vi "Write Ack.vi"(10 "id":u32) -> (2 "channel":T1)   [LabVIEW 2019, in "MessengerM.lvlib"]
doc: "Writes an acknowledgement to a Messenger channel that the message with the given id has been read."
uses:
  <resource>/Channels/MessengerM/MessengerM.lvlib
  <resource>/Channels/MessengerM/EndpointOp.ctl
  <resource>/Channels/MessengerM/ParmsIn.ctl
  <resource>/Channels/MessengerM/))Channel.ctl
  <resource>/Channels/MessengerM/Element.ctl
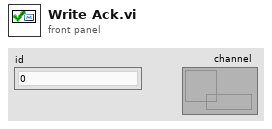
[diagram p1: front panel]
types:
  T1 = typedef "MessengerM.lvlib/))Channel.ctl" = refnum<queue>
  T2 = typedef "MessengerM.lvlib/ParmsIn.ctl" = cluster{"subchannel":i32, "size (0)":i32, "abort (F)":bool, "timeout":i32, "ack id (0)":u32, "last elt? (F)":bool, "valid? (T)":bool, "GUID":string}
  T3 = typedef "MessengerM.lvlib/EndpointOp.ctl" = enum16{"Write", "WriteAck", "WriteSync", "Read", "ReadAck"}
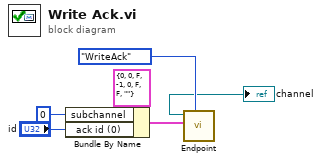
[diagram p0: block diagram]
diagram:
  n1 = Bundle By Name(cluster=T2 {"subchannel"=0, "size (0)"=0, "abort (F)"=FALSE, "timeout"=-1, "ack id (0)"=0, "last elt? (F)"=FALSE, "valid? (T)"=FALSE, "GUID"=""} ("parms in"), "subchannel"=0, "ack id (0)"="id") -> (w3:T2)
  n2 = call <resource>:"Endpoint.vi"("endpointOp"=EndpointOp."WriteAck", "parms in"=w3, "channel in"="channel") -> ()  [unwired: 7 in, 2 out]
